vi "Shooter Auto Selection.vi"() -> ()   [LabVIEW 2019]
panel:
  in  "Hood Setpoint Command":dbl
  in  "Turret Setpoint Command":dbl
  in  "Shooter Setpoint Command":dbl
  in  "Auto-Shot?":bool
  out "Reset Shooter":bool
  out "Reset Hood":bool
  out "Reset Turret":bool
  out "Hood Value":dbl
  out "Turret Value":dbl
  out "Shooter Value":dbl
  in  "Operation Changed?":bool
  in  "cluster":T1
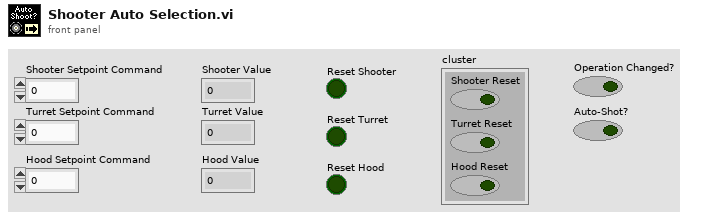
[diagram p1: front panel]
types:
  T1 = cluster{"Shooter Reset":bool, "Turret Reset":bool, "Hood Reset":bool}
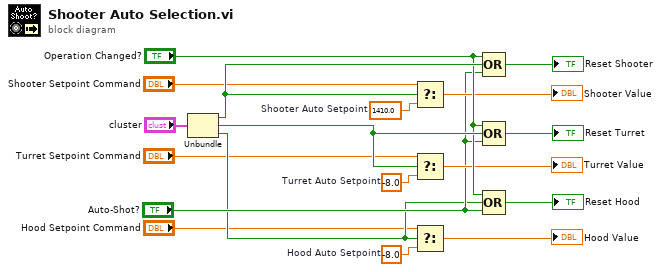
[diagram p0: block diagram]
diagram:
  w13 = -8.0  # Turret Auto Setpoint
  w17 = 1410.0  # Shooter Auto Setpoint
  w18 = -8.0  # Hood Auto Setpoint
  n1 = Unbundle("cluster") -> ("Shooter Reset"=w16:bool, "Turret Reset"=w15:bool, "Hood Reset"=w4:bool)
  n2 = Select(t="Shooter Setpoint Command", s=w16, f=w17) -> (s? t:f=→"Shooter Value":dbl)
  n3 = Select(t="Turret Setpoint Command", s=w15, f=w13) -> (s? t:f=→"Turret Value":dbl)
  n4 = Select(t="Hood Setpoint Command", s=w4, f=w18) -> (s? t:f=→"Hood Value":dbl)
  n5 = Compound Arithmetic op=OR("Operation Changed?", w16, "Auto-Shot?") -> (→"Reset Shooter":bool)
  n6 = Compound Arithmetic op=OR("Operation Changed?", w15, "Auto-Shot?") -> (→"Reset Turret":bool)
  n7 = Compound Arithmetic op=OR("Operation Changed?", w4, "Auto-Shot?") -> (→"Reset Hood":bool)
